vi "Get 1D Time Stamp.vi"(5 "format string (%s)":string="%s", 7 "key description":string, 8 "sections":string[](array[string]), 9 "time stamp":timestamp[](array[timestamp]), 11 "info data":string) -> (0 "sections out":string[](array[string]), 2 "value":timestamp[](array[timestamp]), 3 "info data out":string)   [LabVIEW 2019, in "infolib.lvlib"]
doc: "Reads horizontal or vertical vector of time stamps. If section is entered it searches the key in the section(s)."
uses:
  infolib.lvlib
  Get 2D Time Stamp.vi
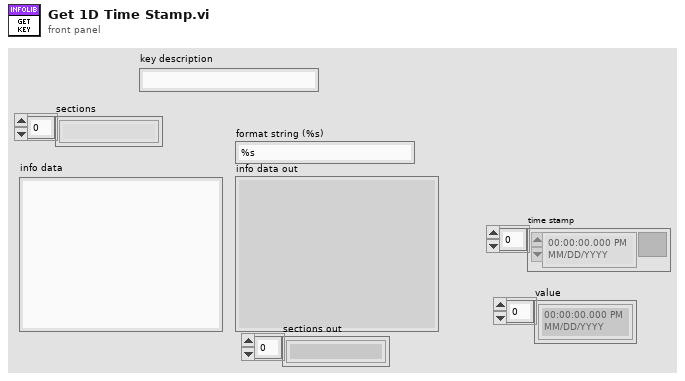
[diagram p1: front panel]
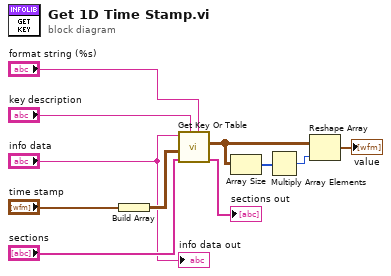
[diagram p0: block diagram]
diagram:
  n1 = Build Array("time stamp") -> (w10:timestamp[][])
  n2 = call-poly "Get Key Or Table.vi"("format string (%s)"="format string (%s)", "key description"="key description", "sections"="sections", "time stamp"=w10, "info data"="info data") -> ("sections out"=→"sections out":string[], "value"=w2:timestamp[][])  [unwired: 4 in, 1 out]
  n3 = Array Size(array=w2) -> (size(s)=w3:i32[])
  n4 = Multiply Array Elements(1:w3) -> (0:w4:i32)
  n5 = Reshape Array(w2, w4) -> (→"value":timestamp[])
  "info data out" <- "info data"
